vi "Read Name.vi"(8 "error in (no error)":errorcluster, 11 "SQS in":refnum<class "SQS.lvclass">) -> (0 "error out":errorcluster, 2 "Name":string, 3 "SQS out":refnum<class "SQS.lvclass">)   [LabVIEW 2015, in "NI_SQS.lvlib" / "SQS.lvclass"]
uses:
  SQS.lvclass
  SQS.lvclass/SQS.ctl
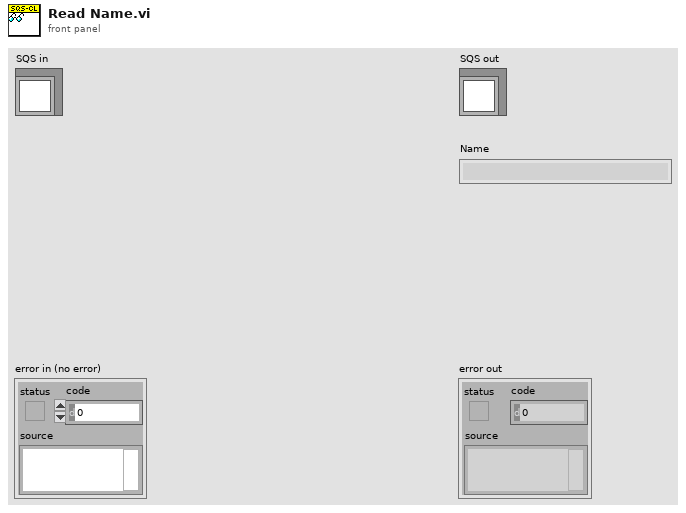
[diagram p1: front panel]
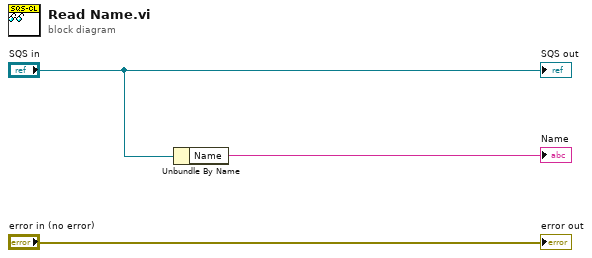
[diagram p0: block diagram]
diagram:
  n1 = Unbundle By Name("SQS in") -> ("Name"=→"Name":string)
  "error out" <- "error in (no error)"
  "SQS out" <- "SQS in"
